vi "set Baud Rate.vi"(10 "baudrate":i32, 11 "port_num":i32) -> (3 "function return":u8)   [LabVIEW 2015, in "dxl_x86_c.lvlib"]
doc: "WINDECLSPEC uint8_t setBaudRate (int port_num, const int baudrate);"
uses:
  dxl_x86_c.lvlib
  dxl_x86_c.dll
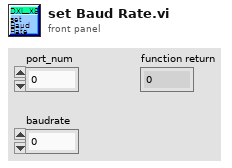
[diagram p1: front panel]
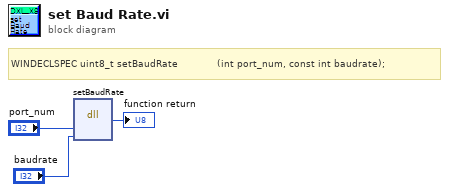
[diagram p0: block diagram]
diagram:
  # "WINDECLSPEC uint8_t setBaudRate             (int port_num, const int baudrate);"
  n1 = dll-call lib="C:/Users/Platform/Desktop/LabVIEW/dxl_x86_c.lvlib/dxl_x86_c.*" fn="setBaudRate"("port_num"="port_num", "baudrate"="baudrate") -> (→"function return":u8)  [unwired: 5 in, 2 out]
